vi "ReadInfo.vi"(8 "error in (no error)":errorcluster, 11 "TCP Network Connection in":refnum<k5>) -> (0 "error out":errorcluster, 1 "Empty?":bool, 2 "output cluster":T1, 3 "TCP Network Connection out":refnum<k5>, 5 "data out 2":string)   [LabVIEW 2013]
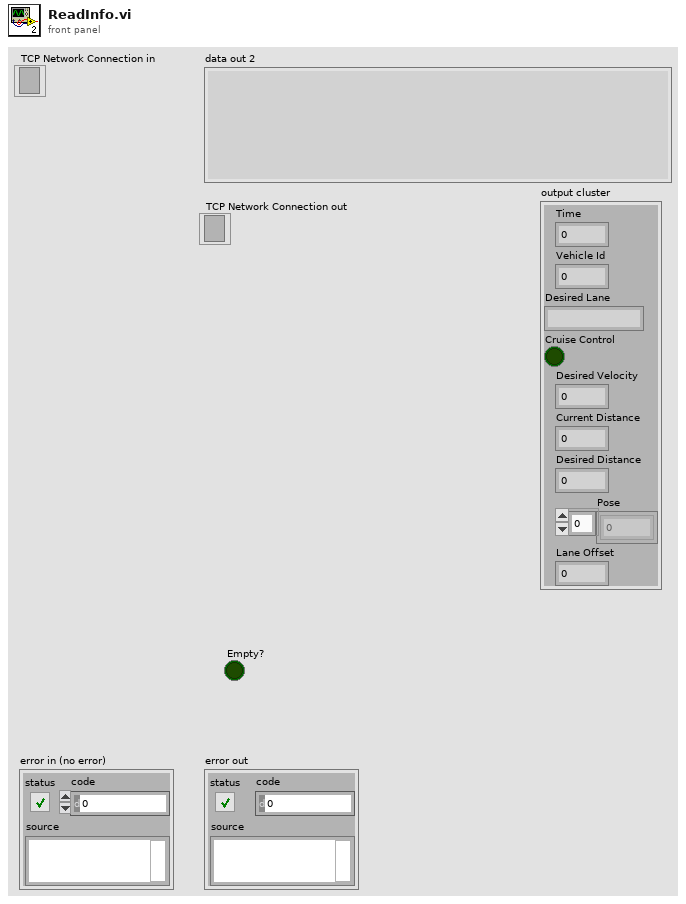
[diagram p1: front panel]
types:
  T1 = cluster{"Time":dbl, "Vehicle Id":i32, "Desired Lane":string, "Cruise Control":bool, "Desired Velocity":dbl, "Current Distance":dbl, "Desired Distance":dbl, "Pose":dbl[], "Lane Offset":dbl}
  T2 = enum16{"Standard", "Buffered", "CRLF", "Immediate"}
  T3 = cluster{"Time":dbl, "Vehicle Id":i32, "Lane":string, "Cruise Control":bool, "Desired Velocity":dbl, "Desired Distance":dbl, "Current Distance":dbl, "X":dbl, "Y":dbl, "Yaw":dbl, "Lane Offset":dbl}
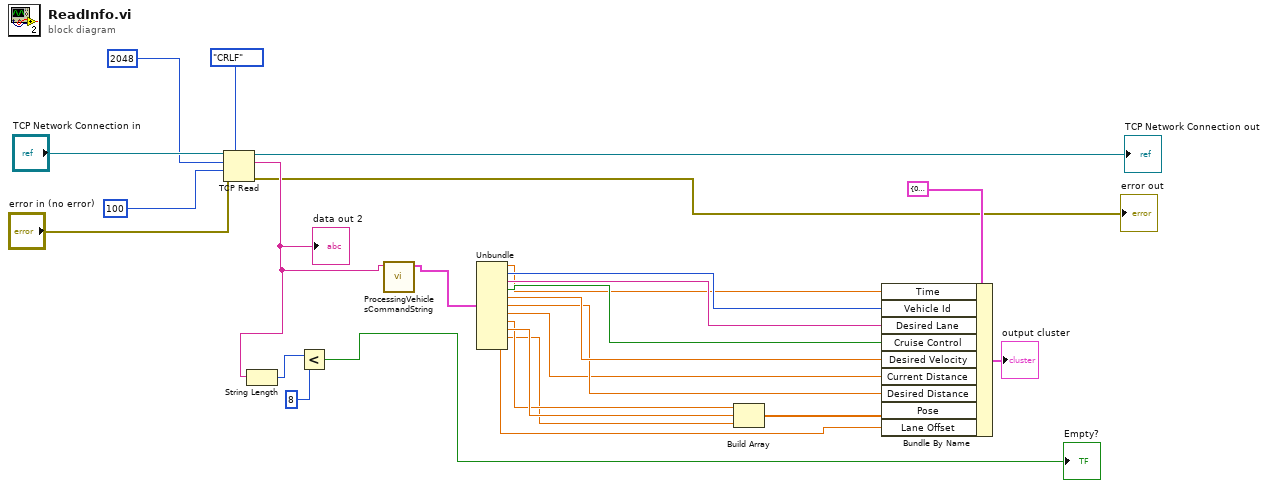
[diagram p0: block diagram]
diagram:
  n1 = TCP Read(connection ID="TCP Network Connection in", bytes to read=2048, error in (no error)="error in (no error)", 7:T2."CRLF" ("mode (standard)"), 9:100 ("timeout ms (25000)")) -> (connection ID out=→"TCP Network Connection out":refnum<k5>, data out=w23:string, error out=→"error out":errorcluster)
  "data out 2" <- w23
  n2 = String Length(string=w23) -> (length=w25:i32)
  n3 = Less?(x=w25, y=8) -> (x < y?=→"Empty?":bool)
  n4 = call "ProcessingVehiclesCommandString.vi"("input string"=w23) -> ("output cluster"=w21:T3)  [unwired: 10 in]
  n5 = Unbundle(w21) -> ("Time"=w16:dbl, "Vehicle Id"=w17:i32, "Lane"=w22:string, "Cruise Control"=w18:bool, "Desired Velocity"=w19:dbl, "Desired Distance"=w5:dbl, "Current Distance"=w4:dbl, "X"=w13:dbl, "Y"=w14:dbl, "Yaw"=w3:dbl, "Lane Offset"=w2:dbl)
  n6 = Build Array(w13, w14, w3) -> (w20:dbl[])
  n7 = Bundle By Name(cluster=T1 {"Time"=0.0, "Vehicle Id"=0, "Desired Lane"="", "Cruise Control"=FALSE, "Desired Velocity"=0.0, "Current Distance"=0.0, "Desired Distance"=0.0, "Pose"=[], "Lane Offset"=0.0} ("Cluster 2"), "Time"=w16, "Vehicle Id"=w17, "Desired Lane"=w22, "Cruise Control"=w18, "Desired Velocity"=w19, "Current Distance"=w4, "Desired Distance"=w5, "Pose"=w20, "Lane Offset"=w2) -> (→"output cluster":T1)
